vi "BRig_dataAnalog_valueAI0_3.vi"() -> (2 "output_valueAI0_3":i32)   [LabVIEW 2014]
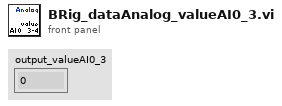
[diagram p1: front panel]
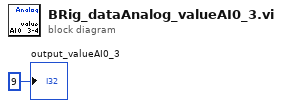
[diagram p0: block diagram]
diagram:
  "output_valueAI0_3" <- 9 ("output_iBlock")
